vi "数据查询_数据查询.vi"() -> ()   [LabVIEW 2016, in "数据查询.lvlib"]
uses:
  <vilib>/Utility/miscctls.llb/LVPointTypeDef.ctl
  <userlib>/_OpenG.lib/array/array.llb/Sort 2D Array (String)__ogtk.vi
  System.Windows.Forms
panel:
  in  "数据类型":string(combo)="N"
  out "columns":string[](array[string])
  out "表格":string[][](table)
  in  "是否剔除异常数据":bool=TRUE
  in  "WebBrowser":refnum<k24>(container)
  in  "列表框":i32(listbox)
  in  "导出":bool
  in  "测量模式":string(combo)="全部数据"
  out "选中数据表":string
  in  "查询":bool
  in  "结束日期":string="2050/01/01"
  in  "起始日期":string="2010/01/01"
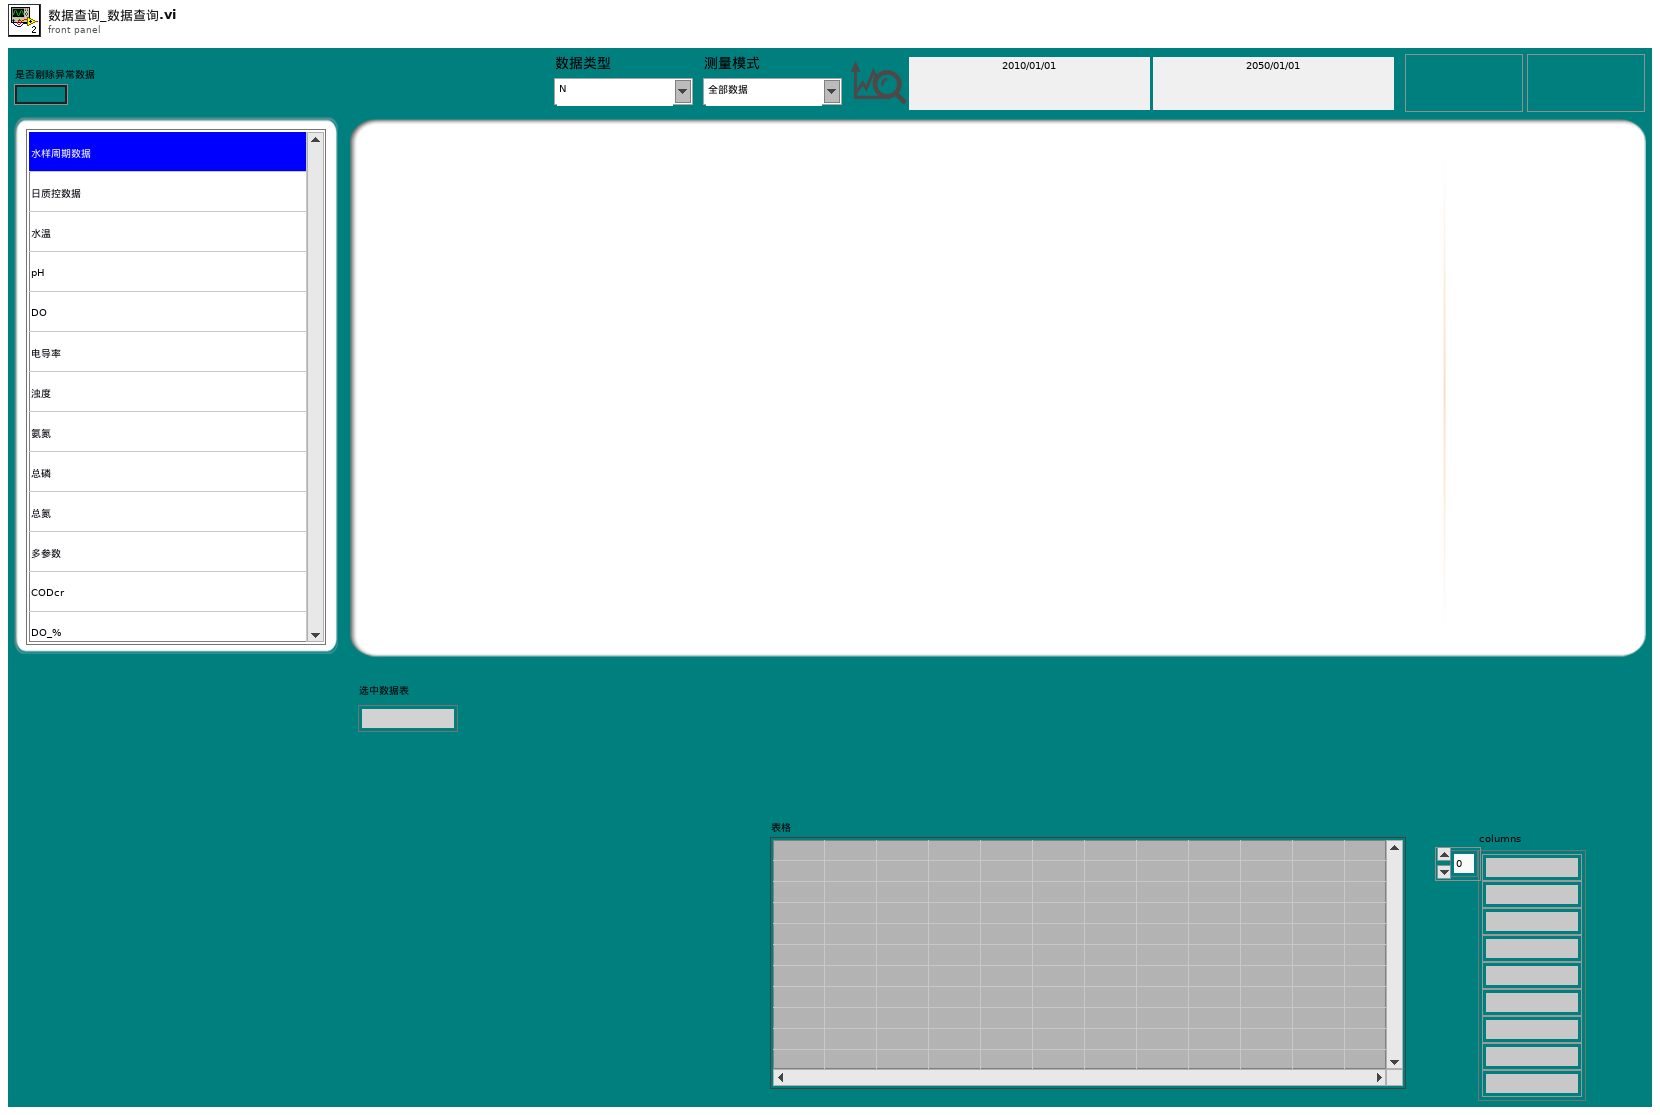
[diagram p1: front panel]
types:
  T1 = typedef "LVPointTypeDef.ctl" = cluster{"Horizontal":i16, "Vertical":i16}
  T2 = typedef "LVDateTimeRec.ctl" = cluster{"秒数的小数部分":dbl, "秒":i32, "分":i32, "时":i32, "日":i32, "月":i32, "年":i32, "天数（周）":i32, "天数（年）":i32, "DST":i32}
  T3 = enum8{"Enabled", "Disabled", "Disabled and Grayed Out"}
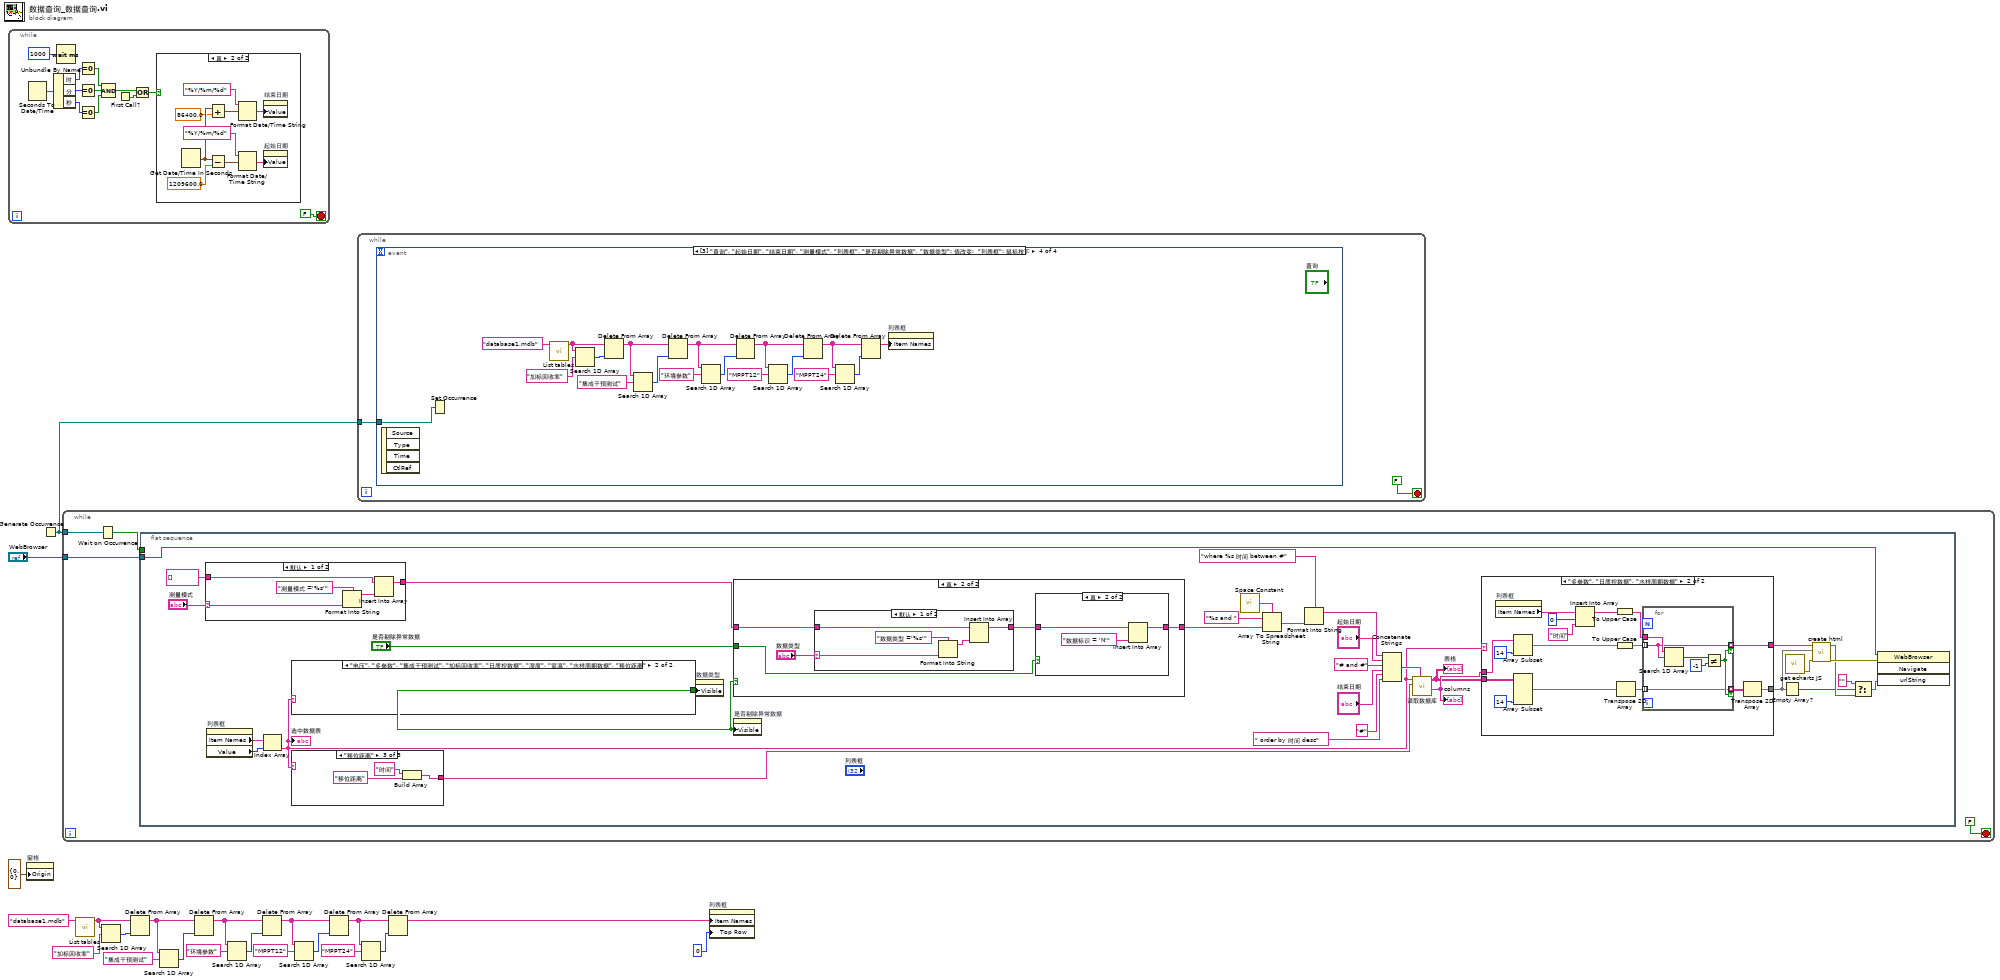
[diagram p0: block diagram]
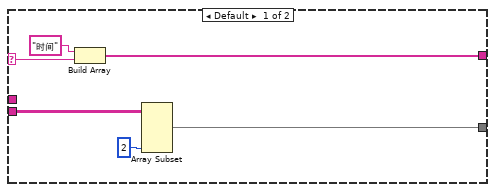
[diagram p6: hidden frame]
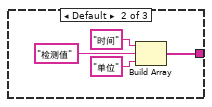
[diagram p8: hidden frame]
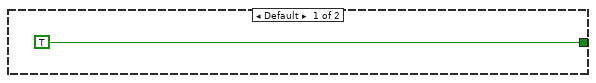
[diagram p9: hidden frame]
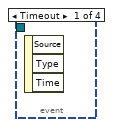
[diagram p11: hidden frame]
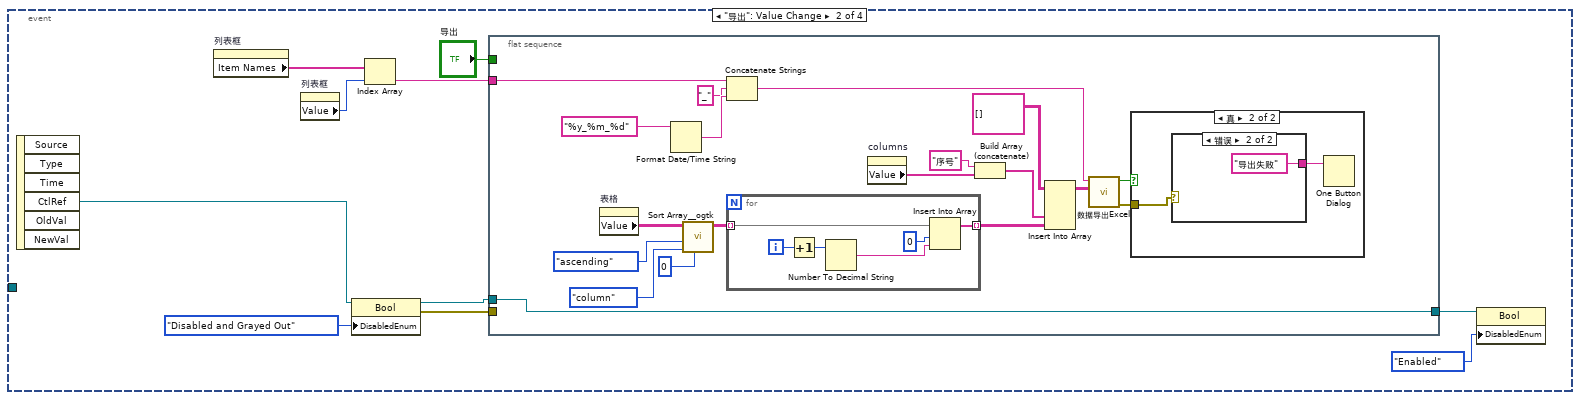
[diagram p12: hidden frame]
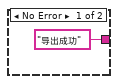
[diagram p14: hidden frame]
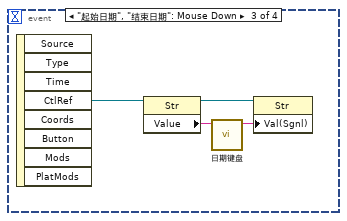
[diagram p15: hidden frame]
diagram:
  n1 = while {
    stop <- FALSE stop-if-true
    n2 = Seconds To Date/Time() -> (date time rec=w33:T2)  [unwired: 2 in]
    n3 = Unbundle By Name(w33) -> ("时"=w32:i32, "分"=w31:i32, "秒"=w30:i32)
    n4 = Wait (ms)(milliseconds to wait=u32 1000 ("等待时间（毫秒）")) -> ()  [unwired: 1 out]
    n5 = Equal To 0?(x=w32) -> (x = 0?=w29:bool)
    n6 = Equal To 0?(x=w31) -> (x = 0?=w28:bool)
    n7 = Equal To 0?(x=w30) -> (x = 0?=w27:bool)
    n8 = Compound Arithmetic op=AND ("复合运算")(w29, w28, w27) -> (w24:bool)
    n9 = First Call?() -> (First Call?: T/F=w22:bool)
    n10 = Or(x=w24, y=w22) -> (x .or. y?=w23:bool)
    n11 = case shown="真" w23 {
      frame False {
      }
      frame True {
        n12 = Get Date/Time In Seconds() -> (seconds since 1Jan1904=w38:timestamp)
        n13 = Add(x=w38, y=86400.0) -> (x+y=w36:timestamp)
        n14 = Subtract(x=w38, y=1209600.0) -> (x-y=w39:timestamp)
        n15 = Format Date/Time String(time format string (%c)="%Y/%m/%d" ("时间格式字符串(%c)"), seconds (now)=w36) -> (date/time string=w35:string)  [unwired: 1 in]
        n16 = Format Date/Time String(time format string (%c)="%Y/%m/%d" ("时间格式字符串(%c)"), seconds (now)=w39) -> (date/time string=w41:string)  [unwired: 1 in]
        n17 = property on="结束日期" class="Str"("Value"=w35) -> ()  [unwired: 2 in, 2 out]
        n18 = property on="起始日期" class="Str"("Value"=w41) -> ()  [unwired: 2 in, 2 out]
      }
    }
  }
  n19 = property on="窗格" class="Pane"("Origin"=T1 {"Horizontal"=0, "Vertical"=0} ("原点")) -> ()  [unwired: 2 in, 2 out]
  n20 = Generate Occurrence() -> (w19:refnum<k4>)
  n21 = while {
    tunnel: w19 -> [w45]
    tunnel: "WebBrowser" -> [w43]
    stop <- FALSE stop-if-true
    n22 = Wait on Occurrence(2:w45) -> (0:w44:bool)  [unwired: 2 in]
    n23 = flat-sequence {
      tunnel: w44 -> [_]
      tunnel: w43 -> [w72]
      frame #0 {
        n24 = case shown="默认" "测量模式" {
          selector: "测量模式" -> [w82 _]
          tunnel: string[] [] -> [w81 w84]
          tunnel: [w79 w84] -> w54
          frame Default {
            n25 = Format Into String(format string="测量模式 ='%s'" ("condition"), w82) -> (resulting string=w80:string)  [unwired: 2 in, 1 out]
            n26 = Insert Into Array(array=w81, new element=w80) -> (w79:string[])  [unwired: 1 in]
          }
          frame "全部数据" {
          }
        }
        n27 = property on="列表框" class="LstBox (严格)"() -> ("Item Names"=w63:string[], "Value"=w62:i32)  [unwired: 2 in, 2 out]
        n28 = Index Array(array=w63, index=w62) -> (element=w66:string)
        "选中数据表" <- w66
        n29 = case shown="\"电压\", \"多参数\", \"集成干预测试\", \"加标回收率\", \"日质控数据\", \"湿度\", \"室温\", \"水样周期数据\", \"移位距离\"" w66 {
          tunnel: [TRUE _] -> w47
          frame Default {
          }
          frame "电压", "多参数", "集成干预测试", "加标回收率", "日质控数据", "湿度", "室温", "水样周期数据", "移位距离" {
          }
        }
        n30 = case shown="\"移位距离\"" w66 {
          tunnel: [_ w129 w133] -> w65
          frame "多参数", "日质控数据", "水样周期数据" {
          }
          frame Default {
            n31 = Build Array("时间", "检测值", "单位" ("元素")) -> (w129:string[])
          }
          frame "移位距离" {
            n32 = Build Array("时间", "移位距离") -> (w133:string[])
          }
        }
        n33 = property on="数据类型" class="CmbBox"("Visible"=w47) -> ()  [unwired: 2 in, 2 out]
        n34 = case shown="真" w47 {
          tunnel: "是否剔除异常数据" -> [_ w90]
          tunnel: w54 -> [w85 w87]
          tunnel: [w85 w86] -> w49
          frame False {
          }
          frame True {
            n35 = case shown="默认" "数据类型" {
              selector: "数据类型" -> [w94 _]
              tunnel: w87 -> [w93 w96]
              tunnel: [w91 w96] -> w88
              frame Default {
                n36 = Format Into String(format string="数据类型 ='%s'" ("condition"), w94) -> (resulting string=w92:string)  [unwired: 2 in, 1 out]
                n37 = Insert Into Array(array=w93, new element=w92) -> (w91:string[])  [unwired: 1 in]
              }
              frame "全部数据" {
              }
            }
            n38 = case shown="真" w90 {
              tunnel: w88 -> [w97 w100]
              tunnel: [w97 w98] -> w86
              frame False {
              }
              frame True {
                n39 = Insert Into Array(array=w100, new element="数据标识 = 'N'" ("condition")) -> (w98:string[])  [unwired: 1 in]
              }
            }
          }
        }
        n40 = property on="是否剔除异常数据" class="Bool (严格)"("Visible"=w47) -> ()  [unwired: 2 in, 2 out]
        n41 = call <vilib>:"Space Constant.vi"() -> ("String"=w52:string)
        n42 = Array To Spreadsheet String(delimiter (Tab)=w52, array=w49, 3:"%s and " ("格式字符串")) -> (spreadsheet string=w53:string)
        n43 = Format Into String(format string="where %s 时间 between #" ("condition"), w53) -> (resulting string=w48:string)  [unwired: 2 in, 1 out]
        n44 = Concatenate Strings(w48, "起始日期", "# and #" ("condition"), "结束日期", "#" ("condition"), " order by 时间 desc" ("字符串")) -> (w78:string)
        n45 = call "读取数据库.vi"("condition"=w78, "显示项"=w65, "组合框"=w66) -> ("columns"=w69:string[], "表格"=w67:string[][])  [unwired: 5 in, 2 out]
        "表格" <- w67
        "columns" <- w69
        n46 = case shown="\"多参数\", \"日质控数据\", \"水样周期数据\"" w66 {
          selector: w66 -> [w103 _]
          tunnel: w69 -> [_ w122]
          tunnel: [w102 w115] -> w68
          tunnel: w67 -> [w106 w120]
          tunnel: [w105 w109] -> w58
          frame Default {
            n47 = Build Array("时间", w103) -> (w102:string[])
            n48 = Array Subset(array=w106, length (col)=2 ("长度")) -> (w105:string[][])  [unwired: 3 in]
          }
          frame "多参数", "日质控数据", "水样周期数据" {
            n49 = property on="列表框" class="LstBox (严格)"() -> ("Item Names"=w112:string[])  [unwired: 2 in, 2 out]
            n50 = Array Subset(array=w122, length=14 ("长度")) -> (w116:string[])  [unwired: 1 in]
            n51 = Array Subset(array=w120, length (col)=14 ("长度")) -> (w114:string[][])  [unwired: 3 in]
            n52 = Insert Into Array(array=w112, index=0 ("索引"), new element="时间" ("新元素/子数组")) -> (w113:string[])
            n53 = To Upper Case(1:w113) -> (0:w107:string[])
            n54 = To Upper Case(1:w116) -> (0:w108:string[])
            n55 = Transpose 2D Array(2D array=w114) -> (transposed array=w118:string[][])
            n56 = for {
              tunnel: w108 -> [w127] mode=indexing
              tunnel: w118 -> [w123] mode=indexing
              tunnel: w107 -> [w128]
              tunnel: [w127] -> w115 mode=indexing if=w124
              tunnel: [w123] -> w117 mode=indexing if=w124
              n57 = Search 1D Array(1D array=w128, element=w127) -> (index of element=w125:i32)  [unwired: 1 in]
              n58 = Not Equal?(x=w125, y=-1) -> (x != y?=w124:bool)
            }
            n59 = Transpose 2D Array(2D array=w117) -> (transposed array=w109:string[][])
          }
        }
        n60 = Empty Array?(array=w58) -> (empty?=w57:bool)
        n61 = call "get echarts JS.vi"() -> ("error out"=w71:errorcluster)  [unwired: 11 in]
        n62 = call "create html.vi"("error in (no error)"=w71, "data"=w58, "columns"=w68) -> ("error out"=w70:errorcluster, "url"=w61:string)  [unwired: 7 in]
        n63 = Select(t="", s=w57, f=w61) -> (s? t:f=w60:string)
        n64 = invoke class="WebBrowser" method="Navigate"(reference=w72, error in=w70, "urlString"=w60) -> ()  [unwired: 1 in, 4 out]
      }
    }
  }
  n65 = call "List tables.vi"("database"="database1.mdb") -> ("tables"=w14:string[])  [unwired: 9 in, 1 out]
  n66 = Search 1D Array(1D array=w14, element="加标回收率" ("元素")) -> (index of element=w13:i32)  [unwired: 1 in]
  n67 = Delete From Array(array=w14, index=w13) -> (array with subset deleted=w11:string[])  [unwired: 1 in, 1 out]
  n68 = Search 1D Array(1D array=w11, element="集成干预测试" ("元素")) -> (index of element=w12:i32)  [unwired: 1 in]
  n69 = Delete From Array(array=w11, index=w12) -> (array with subset deleted=w8:string[])  [unwired: 1 in, 1 out]
  n70 = Search 1D Array(1D array=w8, element="环境参数" ("元素")) -> (index of element=w10:i32)  [unwired: 1 in]
  n71 = Delete From Array(array=w8, index=w10) -> (array with subset deleted=w5:string[])  [unwired: 1 in, 1 out]
  n72 = Search 1D Array(1D array=w5, element="MPPT12" ("元素")) -> (index of element=w6:i32)  [unwired: 1 in]
  n73 = Delete From Array(array=w5, index=w6) -> (array with subset deleted=w2:string[])  [unwired: 1 in, 1 out]
  n74 = while {
    tunnel: w19 -> [w137]
    stop <- FALSE stop-if-true
    n75 = event shown="[3] \"查询\", \"起始日期\", \"结束日期\", \"测量模式\", \"列表框\", \"是否剔除异常数据\", \"数据类型\": 值改变;  \"列表框\": 鼠标按下" {
      selector: _ -> [_ _ _ _]
      dyn-events: _ -> [_ _ _ _]
      timeout: _ -> [_ _ _ _]
      tunnel: w137 -> [_ _ _ w199]
      event Timeout {
        n76 = event-data() -> ()  [unwired: 1 in, 3 out]
      }
      event "导出": Value Change {
        n77 = event-data() -> ("CtlRef"=w148:refnum<vi>)  [unwired: 1 in, 5 out]
        n78 = property on="列表框" class="LstBox (严格)"() -> ("Item Names"=w141:string[])  [unwired: 2 in, 2 out]
        n79 = property on="列表框" class="LstBox (严格)"() -> ("Value"=w140:i32)  [unwired: 2 in, 2 out]
        n80 = property class="Bool"(reference=w148, "DisabledEnum"=T3."Disabled and Grayed Out" ("禁用")) -> (reference out=w145:refnum<vi>, error out=w146:errorcluster)  [unwired: 1 in]
        n81 = Index Array(array=w141, index=w140) -> (element=w139:string)
        n82 = flat-sequence {
          tunnel: w146 -> [_]
          tunnel: [w164] -> w144
          tunnel: w145 -> [w164]
          tunnel: "导出" -> [_]
          tunnel: w139 -> [w154]
          frame #0 {
            n83 = property on="表格" class="Tbl (严格)"() -> ("Value"=w150:string[][])  [unwired: 2 in, 2 out]
            n84 = Format Date/Time String(time format string (%c)="%y_%m_%d" ("时间格式字符串(%c)")) -> (date/time string=w161:string)  [unwired: 2 in]
            n85 = call-poly <userlib>:"Sort Array__ogtk.vi"("Column/Row to Sort By"=u32 0, "Sort By in"=enum16{"row", "column"}."column", "Order"=enum16{"ascending", "descending"}."ascending", "Array in"=w150) -> ("Sorted Array out"=w158:string[][])  [unwired: 4 in, 3 out]
            n86 = Concatenate Strings(w154, "_" ("字符串"), w161) -> (w159:string)
            n87 = for {
              tunnel: w158 -> [w176] mode=indexing
              tunnel: [w175] -> w151 mode=indexing
              i -> [w177]
              n88 = Increment(x=w177) -> (x+1=w173:i32)
              n89 = Number To Decimal String(number=w173) -> (decimal integer string=w172:string)  [unwired: 1 in]
              n90 = Insert Into Array(array=w176, index=0 ("索引"), new element=w172) -> (w175:string[])
            }
            n91 = property on="columns" class="Arr (严格)"() -> ("Value"=w149:string[])  [unwired: 2 in, 2 out]
            n92 = Build Array (concatenate)("序号" ("新元素/子数组"), w149) -> (w152:string[])
            n93 = Insert Into Array(array=string[][] [], new element #1=w152, new element #2=w151) -> (w157:string[][])  [unwired: 2 in]
            n94 = call "数据导出Excel.vi"("text data"=w157, "default name"=w159) -> ("error out"=w156:errorcluster, "布尔"=w155:bool)  [unwired: 8 in]
            n95 = case shown="真" w155 {
              tunnel: w156 -> [_ w169]
              frame False {
              }
              frame True {
                n96 = case shown="错误" w169 {
                  tunnel: ["导出成功" ("消息") "导出失败" ("消息")] -> w168
                  frame No Error {
                  }
                  frame Error {
                  }
                }
                n97 = One Button Dialog(message=w168) -> ()  [unwired: 1 in, 1 out]
              }
            }
          }
        }
        n98 = property class="Bool"(reference=w144, "DisabledEnum"=T3."Enabled" ("禁用")) -> ()  [unwired: 1 in, 2 out]
      }
      event "起始日期", "结束日期": Mouse Down {
        n99 = event-data() -> ("CtlRef"=w181:refnum<vi>)  [unwired: 1 in, 7 out]
        n100 = property class="Str"(reference=w181) -> (reference out=w179:refnum<vi>, "Value"=w180:string)  [unwired: 1 in, 1 out]
        n101 = call "日期键盘.vi"("原值"=w180) -> ("x+y"=w178:string)  [unwired: 10 in]
        n102 = property class="Str"(reference=w179, "Val(Sgnl)"=w178) -> ()  [unwired: 1 in, 2 out]
      }
      event "查询", "起始日期", "结束日期", "测量模式", "列表框", "是否剔除异常数据", "数据类型": Value Change; "列表框": Mouse Down {
        n103 = event-data() -> ()  [unwired: 1 in, 4 out]
        n104 = Set Occurrence(w199) -> ()
        n105 = call "List tables.vi"("database"="database1.mdb") -> ("tables"=w185:string[])  [unwired: 9 in, 1 out]
        n106 = Search 1D Array(1D array=w185, element="加标回收率" ("元素")) -> (index of element=w186:i32)  [unwired: 1 in]
        n107 = Delete From Array(array=w185, index=w186) -> (array with subset deleted=w188:string[])  [unwired: 1 in, 1 out]
        n108 = Search 1D Array(1D array=w188, element="集成干预测试" ("元素")) -> (index of element=w187:i32)  [unwired: 1 in]
        n109 = Delete From Array(array=w188, index=w187) -> (array with subset deleted=w191:string[])  [unwired: 1 in, 1 out]
        n110 = Search 1D Array(1D array=w191, element="环境参数" ("元素")) -> (index of element=w189:i32)  [unwired: 1 in]
        n111 = Delete From Array(array=w191, index=w189) -> (array with subset deleted=w194:string[])  [unwired: 1 in, 1 out]
        n112 = Search 1D Array(1D array=w194, element="MPPT12" ("元素")) -> (index of element=w193:i32)  [unwired: 1 in]
        n113 = Delete From Array(array=w194, index=w193) -> (array with subset deleted=w197:string[])  [unwired: 1 in, 1 out]
        n114 = Search 1D Array(1D array=w197, element="MPPT24" ("元素")) -> (index of element=w195:i32)  [unwired: 1 in]
        n115 = Delete From Array(array=w197, index=w195) -> (array with subset deleted=w198:string[])  [unwired: 1 in, 1 out]
        n116 = property on="列表框" class="LstBox (严格)"("Item Names"=w198) -> ()  [unwired: 2 in, 2 out]
      }
    }
  }
  n117 = Search 1D Array(1D array=w2, element="MPPT24" ("元素")) -> (index of element=w4:i32)  [unwired: 1 in]
  n118 = Delete From Array(array=w2, index=w4) -> (array with subset deleted=w1:string[])  [unwired: 1 in, 1 out]
  n119 = property on="列表框" class="LstBox (严格)"("Item Names"=w1, "Top Row"=0 ("顶行")) -> ()  [unwired: 2 in, 2 out]
